vi "labviewProgram.vi"() -> ()   [LabVIEW 2023]
uses:
  <vilib>/Analysis/3filter.llb/Elliptic Filter (DBL).vi
  <vilib>/Utility/file.llb/Write Delimited Spreadsheet (DBL).vi
  <instrlib>/Ocean Optics 2000 4000/Ocean Optics 2000 4000.lvlib
  <vilib>/Analysis/NI_AAL_SigProc.lvlib
  <vilib>/Analysis/NI_AALBase.lvlib
panel:
  out "波谷/待测量":dbl[][](array[numeric])
  in  "特征值":dbl[](array[numeric])
  in  "?":bool
  out "Locations":dbl[](array[numeric]) caption="位置"
  out "波谷个数":i32 caption="找到波谷个数"
  in  "peaks/valleys":enum32{"Peaks", "Valleys"}(ring) caption="波峰/波谷"
  in  "波谷检测宽度":u32=6000
  in  "滤波器阶数":u32=6000
  out "背景光谱 2":cluster{dbl[], dbl[]}(graph)
  in  "?":bool
  in  "保存文件路径":path
  out "初始光谱":cluster{dbl[], dbl[]}(graph)
  in  "积分时间 (6000us)":u32=6000
  in  "?":dbl=2850.0
  out "光谱":T1(graph)
  in  "Stop":bool
  in  "transmission模式":u16(ring) items=["Absorbance", "Transmission"]
  in  "读取反射光":bool
  in  "读取背景光":bool
  in  "仪器名称":refnum<visa-resource-name>
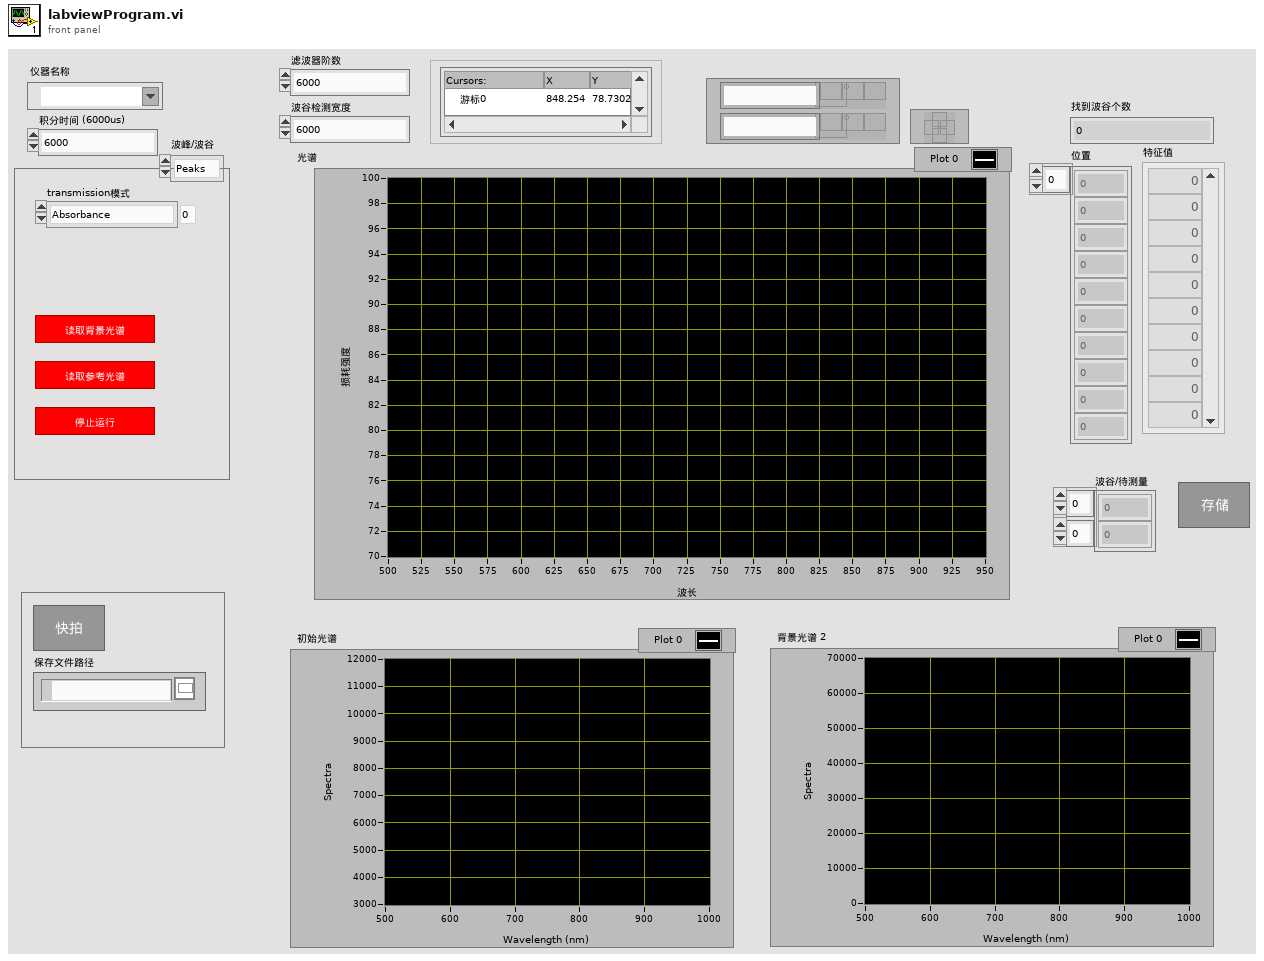
[diagram p1: front panel]
types:
  T1 = cluster{"Wavelength (nm)":dbl[], "Processed Spectrum":dbl[]}
  T2 = cluster{"Wavelength (nm)":dbl[], "Spectrum by Pixel Number":dbl[]}
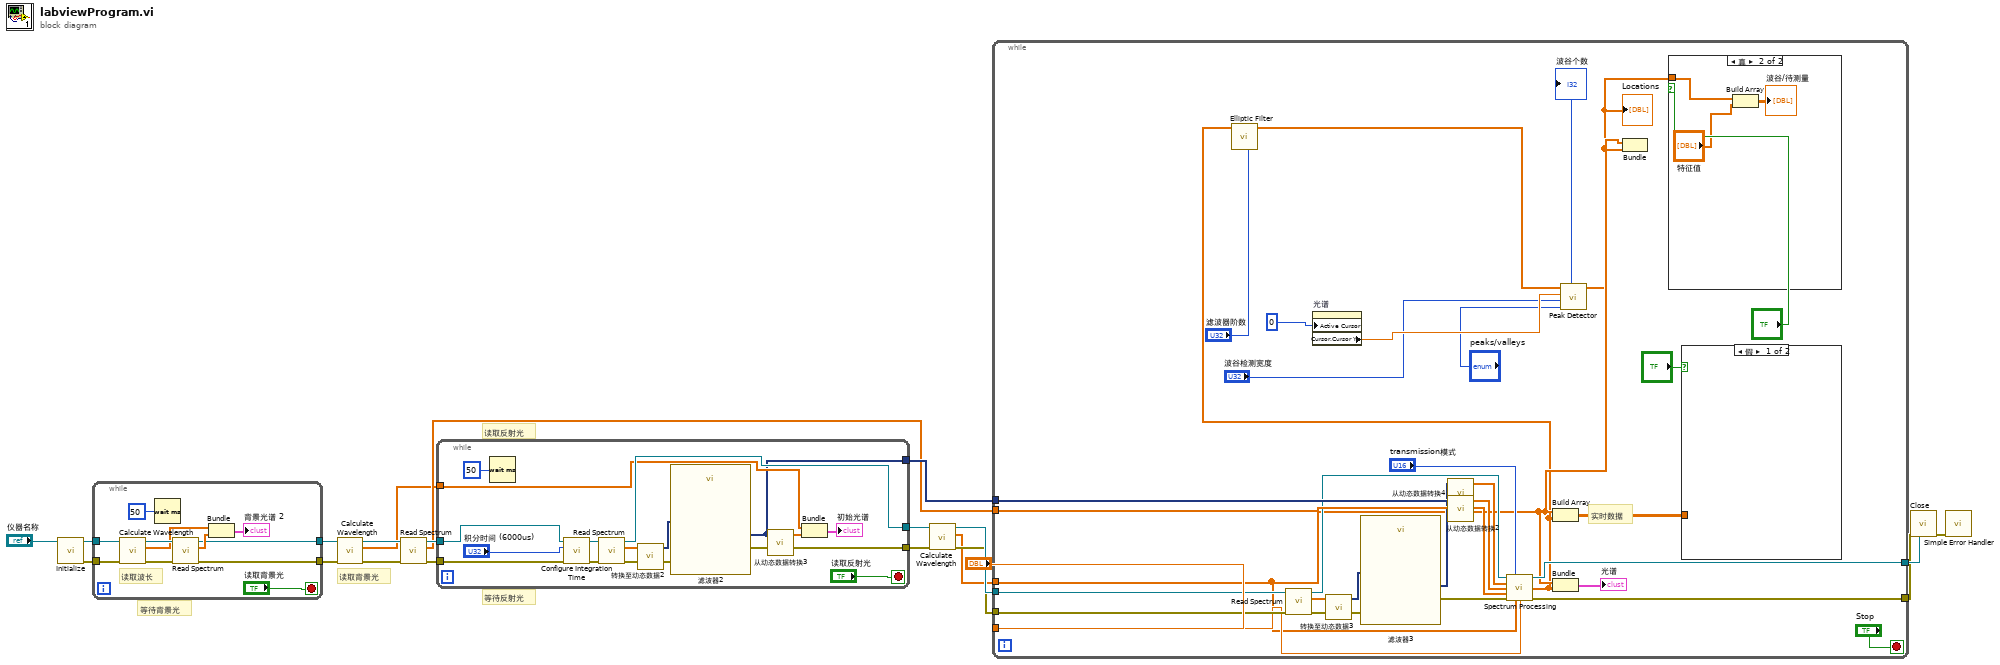
[diagram p0: block diagram]
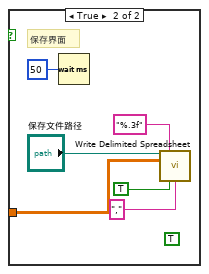
[diagram p3: hidden frame]
diagram:
  # "读取反射光"
  # "读取背景光"
  # "等待反射光"
  # "等待背景光"
  n1 = call <instrlib>:"Initialize.vi"("VISA resource name"="仪器名称") -> ("error out"=w19:errorcluster, "VISA resource name out"=w20:refnum<visa-resource-name>)  [unwired: 2 in, 7 out]
  n2 = while {
    tunnel: [w22] -> w12
    tunnel: w20 -> [w23]
    tunnel: [w24] -> w9
    tunnel: w19 -> [w25]
    stop <- "读取背景光" stop-if-true
    # "读取波长"
    n3 = call <instrlib>:"Calculate Wavelength.vi"("error in (no error)"=w25, "VISA resource name"=w23) -> ("error out"=w30:errorcluster, "Wavelength (nm)"=w28:dbl[], "VISA resource name out"=w29:refnum<visa-resource-name>)  [unwired: 1 in, 6 out]
    n4 = Wait (ms)(milliseconds to wait=u32 50 ("millisecond multiple")) -> ()  [unwired: 1 out]
    n5 = call <instrlib>:"Read Spectrum.vi"("error in (no error)"=w30, "VISA resource name"=w29) -> ("error out"=w24:errorcluster, "Spectrum by Pixel Number"=w27:dbl[], "VISA resource name out"=w22:refnum<visa-resource-name>)  [unwired: 6 in, 1 out]
    n6 = Bundle("Wavelength (nm)"=w28, "Spectrum by Pixel Number"=w27) -> (→"背景光谱 2":T2)  [unwired: 1 in]
  }
  n7 = call <instrlib>:"Calculate Wavelength.vi"("error in (no error)"=w9, "VISA resource name"=w12) -> ("error out"=w10:errorcluster, "Wavelength (nm)"=w1:dbl[], "VISA resource name out"=w11:refnum<visa-resource-name>)  [unwired: 1 in, 6 out]
  n8 = call <instrlib>:"Read Spectrum.vi"("error in (no error)"=w10, "VISA resource name"=w11) -> ("error out"=w5:errorcluster, "Spectrum by Pixel Number"=w2:dbl[], "VISA resource name out"=w6:refnum<visa-resource-name>)  [unwired: 6 in, 1 out]
  n9 = while {
    tunnel: w6 -> [w43]
    tunnel: [w37] -> w7
    tunnel: w5 -> [w42]
    tunnel: [w41] -> w4
    tunnel: [w34] -> w3
    tunnel: w1 -> [w40]
    stop <- "读取反射光" stop-if-true
    n10 = Wait (ms)(milliseconds to wait=u32 50 ("millisecond multiple")) -> ()  [unwired: 1 out]
    n11 = call <instrlib>:"Configure Integration Time.vi"("error in (no error)"=w42, "Integration Time (6000)"="积分时间 (6000us)", "VISA resource name"=w43) -> ("error out"=w45:errorcluster, "VISA resource name out"=w44:refnum<visa-resource-name>)  [unwired: 7 in]
    n12 = call <instrlib>:"Read Spectrum.vi"("error in (no error)"=w45, "VISA resource name"=w44) -> ("error out"=w38:errorcluster, "Spectrum by Pixel Number"=w36:dbl[], "VISA resource name out"=w41:refnum<visa-resource-name>)  [unwired: 6 in, 1 out]
    n13 = call "转换至动态数据2"("Array"=w36) -> ("Dynamic Data Type"=w35:dynamicdata)  [unwired: 3 in]
    n14 = call "滤波器2"("error in (no error)"=w38, "Signal"=w35) -> ("error out"=w37:errorcluster, "Filtered Signal"=w34:dynamicdata)  [unwired: 8 in]
    n15 = call "从动态数据转换3"("Dynamic Data Type"=w34) -> ("Array"=w33:dbl[])  [unwired: 3 in]
    n16 = Bundle("Wavelength (nm)"=w40, "Array"=w33) -> (→"初始光谱":cluster{"Wavelength (nm)":dbl[], "Array":dbl[]})  [unwired: 1 in]
  }
  n17 = call <instrlib>:"Calculate Wavelength.vi"("error in (no error)"=w7, "VISA resource name"=w4) -> ("error out"=w17:errorcluster, "Wavelength (nm)"=w8:dbl[], "VISA resource name out"=w18:refnum<visa-resource-name>)  [unwired: 1 in, 6 out]
  n18 = while {
    tunnel: w2 -> [w79]
    tunnel: w3 -> [w78]
    tunnel: w18 -> [w76]
    tunnel: w17 -> [w77]
    tunnel: w8 -> [w54]
    tunnel: "?" -> [w74]
    tunnel: [w73] -> w15
    tunnel: [w72] -> w14
    stop <- "Stop" stop-if-true
    # "实时数据"
    n19 = call <instrlib>:"Read Spectrum.vi"("error in (no error)"=w77, "VISA resource name"=w76) -> ("error out"=w62:errorcluster, "Spectrum by Pixel Number"=w66:dbl[], "VISA resource name out"=w75:refnum<visa-resource-name>)  [unwired: 6 in, 1 out]
    n20 = property on="光谱" class="XYGraph (严格)"("Active Cursor"=u32 0 ("活动游标")) -> ("Cursor.Cursor Y"=w59:dbl)  [unwired: 2 in, 2 out]
    n21 = call "转换至动态数据3"("Array"=w66) -> ("Dynamic Data Type"=w65:dynamicdata)  [unwired: 3 in]
    n22 = call "滤波器3"("error in (no error)"=w62, "Signal"=w65) -> ("error out"=w61:errorcluster, "Filtered Signal"=w64:dynamicdata)  [unwired: 8 in]
    n23 = call "从动态数据转换4"("Dynamic Data Type"=w64) -> ("Array"=w63:dbl[])  [unwired: 3 in]
    n24 = call "从动态数据转换2"("Dynamic Data Type"=w78) -> ("Array"=w67:dbl[])  [unwired: 3 in]
    n25 = call <instrlib>:"Spectrum Processing.vi"("VISA resource name"=w75, "Spectral Mode (0:Absorbance)"="transmission模式", "Sample Spectrum"=w63, "Reference Spectrum"=w67, "Dark Spectrum"=w79, "error in (no error)"=w61, "Wavelength (nm)"=w54, "Color Temperature (2850 K)"=w74) -> ("VISA resource name out"=w73:refnum<visa-resource-name>, "Processed Spectrum"=w49:dbl[], "error out"=w72:errorcluster)  [unwired: 5 out]
    n26 = call-poly <vilib>:"Elliptic Filter.vi"("order"="滤波器阶数", "X"=w49) -> ("Filtered X"=w60:dbl[])  [unwired: 8 in, 1 out]
    n27 = Build Array(w54, w49) -> (w69:dbl[][])
    n28 = Bundle("Wavelength (nm)"=w54, "Processed Spectrum"=w49) -> (→"光谱":T1)  [unwired: 1 out]
    n29 = call <vilib>:"Peak Detector.vi"("peaks/valleys"="peaks/valleys", "width"="波谷检测宽度", "threshold"=w59, "X"=w60) -> ("Locations"=w50:dbl[], "# found"=→"波谷个数":i32)  [unwired: 3 in, 3 out]
    "Locations" <- w50
    n30 = Bundle("Wavelength (nm)"=w54, "Locations"=w50) -> ()  [unwired: 2 out]
    n31 = case shown="真" "?" {
      tunnel: w50 -> [_ w82]
      frame False {
      }
      frame True {
        n32 = Build Array(w82, "特征值") -> (→"波谷/待测量":dbl[][])
      }
    }
    n33 = case shown="假" "?" {
      tunnel: w69 -> [_ w87]
      frame False {
      }
      frame True {
        (unwired) TRUE ("append to file? (new file:F)")
        # "保存界面"
        n34 = Wait (ms)(milliseconds to wait=u32 50 ("millisecond multiple")) -> ()  [unwired: 1 out]
        n35 = call-poly <vilib>:"Write Delimited Spreadsheet.vi"("file path (dialog if empty)"="保存文件路径", "format (%.3f)"="%.3f", "2D data"=w87, "transpose? (no:F)"=TRUE, "delimiter (\\t)"=",") -> ()  [unwired: 9 in, 2 out]
      }
    }
  }
  n36 = call <instrlib>:"Close.vi"("error in (no error)"=w14, "VISA resource name"=w15) -> ("error out"=w13:errorcluster)  [unwired: 9 out]
  n37 = call <vilib>:"Simple Error Handler.vi"("error in (no error)"=w13) -> ()  [unwired: 1 in, 8 out]
